vi "System Semaphore Create.vi"(8 "error in (no error)":errorcluster, 9 "MaximumCount":i32=1, 10 "Initial Count":i32=1, 11 "Name":string="LabVIEW_System_Semaphore") -> (0 "error out":errorcluster, 3 "Handle":u16 format="%.0x")   [LabVIEW 2011]
uses:
  kernel32.dll
panel:
  out "maximumCount":i32
  out "initalCount":i32
  out "name":string
  out "output param":T1
  # "Returns Handle to a Named System Semaphore, \nor Creates it if it does not exist."
  # "Semaphore is locked when Count reaches 0"
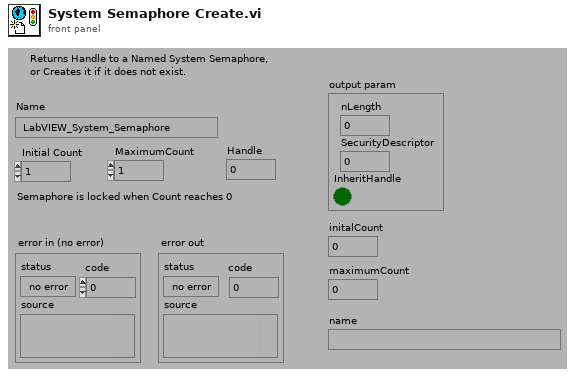
[diagram p1: front panel]
types:
  T1 = cluster{"nLength":u16, "SecurityDescriptor":i32, "InheritHandle":bool}
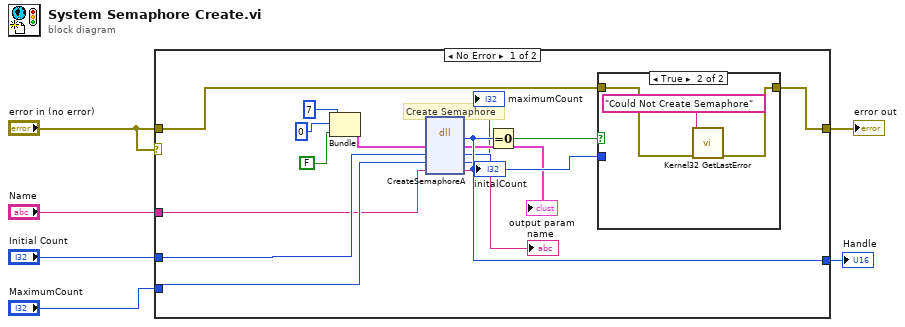
[diagram p0: block diagram]
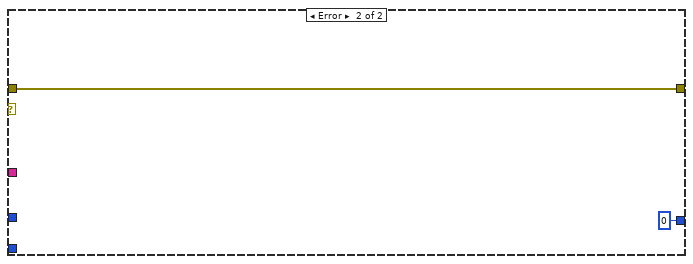
[diagram p3: hidden frame]
diagram:
  n1 = case shown="No Error" "error in (no error)" {
    tunnel: "error in (no error)" -> [w15 w27]
    tunnel: [w14 w27] -> w3
    tunnel: "Name" -> [w16 _]
    tunnel: "Initial Count" -> [w21 _]
    tunnel: "MaximumCount" -> [w20 _]
    tunnel: [w12 0] -> w2
    frame No Error {
      # "Create Semaphore"
      n2 = Bundle("nLength"=u16 7, "SecurityDescriptor"=0, "InheritHandle"=FALSE) -> (w11:T1)  [unwired: 1 in]
      n3 = dll-call lib="kernel32.dll" fn="CreateSemaphoreA"("output param"=w11, "initalCount"=w21, "maximumCount"=w20, "name"=w16) -> (w12:u16, "output param"=→"output param":T1, "initalCount"=→"initalCount":i32, "maximumCount"=→"maximumCount":i32, "name"=→"name":string)  [unwired: 3 in, 2 out]
      n4 = Equal To 0?(x=w12) -> (x = 0?=w13:bool)
      n5 = case shown="True" w13 {
        tunnel: w15 -> [w22 w23]
        tunnel: [w22 w25] -> w14
        tunnel: w12 -> [_ _]
        frame False {
          # "No Error"
        }
        frame True {
          n6 = call "Kernel32 GetLastError.vi"("error in (no error)"=w23, "Message"="Could Not Create Semaphore" ("source")) -> ("error out"=w25:errorcluster)  [unwired: 9 in]
        }
      }
    }
    frame Error {
      (unwired) FALSE
    }
  }
  "error out" <- w3
  "Handle" <- w2
